vi "Match idot to shot.vi"(8 "error in (no error)":errorcluster, 10 "Idot match record":T1, 11 "Cap Bank Server in":refnum<class "Cap Bank Server.lvclass">) -> (0 "error out":errorcluster, 3 "Cap Bank Server out":refnum<class "Cap Bank Server.lvclass">)   [LabVIEW 2015, in "Cap Bank Server.lvclass"]
uses:
  Cap Bank Server.lvclass
  Idot match record.ctl
  <vilib>/ActorFramework/Actor/Actor.lvclass/Actor.ctl
  <vilib>/ActorFramework/Message Enqueuer/Message Enqueuer.lvclass/Message Enqueuer.ctl
  Mag Lab Measure Controller Messages/Log Status Update Msg/Log Status Update Msg.lvclass/Log Status Update Msg.ctl
  Cap Bank Server Messages/Match idot to shot Msg/Match idot to shot Msg.lvclass/Match idot to shot Msg.ctl
  <vilib>/ActorFramework/Message Enqueuer/Init from Existing Queue.vi
  <vilib>/ActorFramework/Message Enqueuer/Enqueue.vi
  <vilib>/ActorFramework/Message Priority Queue/Priority Enqueue.vi
  <vilib>/ActorFramework/Time-Delayed Send Message/Time-Delayed Send Message.vi
  <vilib>/ActorFramework/Message Enqueuer/Message Enqueuer.lvclass
  Mag Lab Measure Controller Messages/Log Status Update Msg/Log Status Update Msg.lvclass
  Cap Bank Server Messages/Match idot to shot Msg/Match idot to shot Msg.lvclass
  <vilib>/ActorFramework/Actor/Actor.lvclass
  Mag Lab Error Handler/Mag Lab Error Handler.lvclass
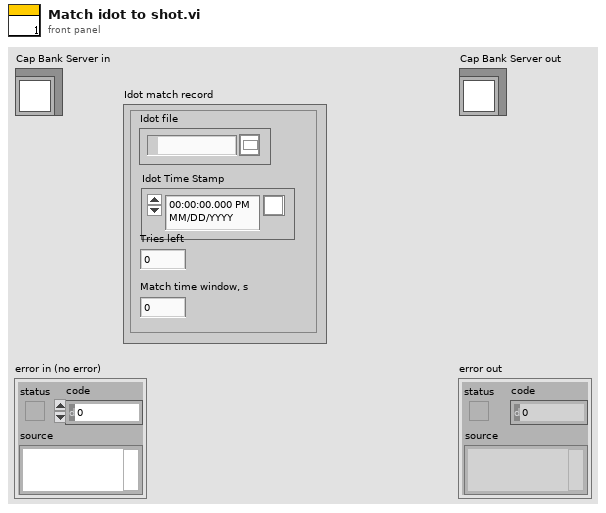
[diagram p1: front panel]
types:
  T1 = typedef "Idot match record.ctl" = cluster{"Idot file":path, "Idot Time Stamp":timestamp, "Tries left":i32, "Match time window, s":dbl}
  T2 = typedef "Shot data.ctl" = cluster{"Shot number":i32, "Time":timestamp, "Magnet ID":string, "User":string, "Cell number":i32, "Requested field":dbl, "Field direction":string, "Number of bank frames":i32, "Crowbar resistance, mOhm":dbl, "Magnet resistance, mOhm":dbl, "Charger voltage, kV":dbl, "Frame voltage, kV":dbl}
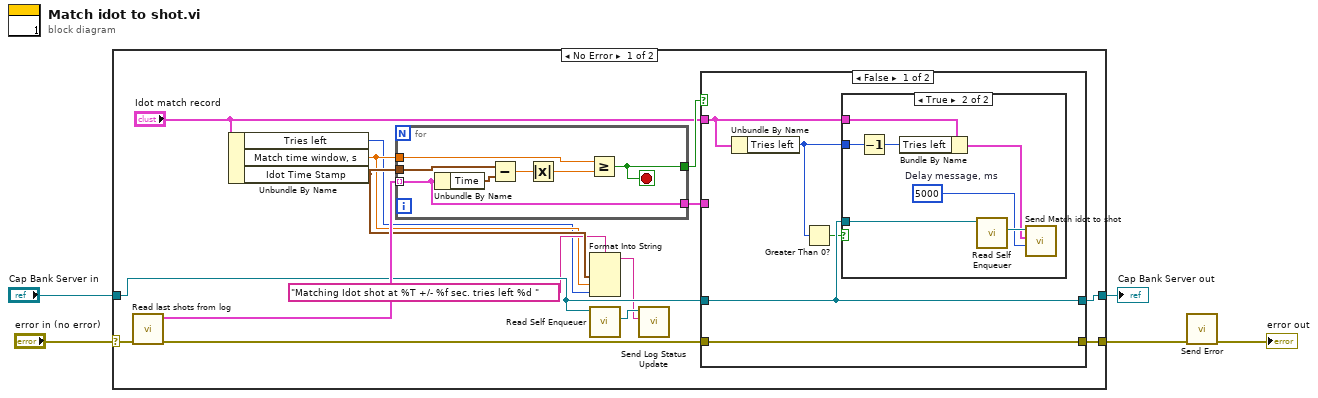
[diagram p0: block diagram]
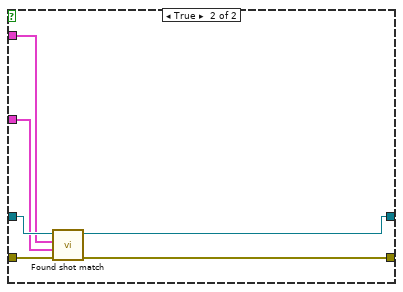
[diagram p3: hidden frame]
diagram:
  n1 = case shown="No Error" "error in (no error)" {
    selector: "error in (no error)" -> [w19 w47]
    tunnel: [w16 w47] -> w2
    tunnel: [w15 w46] -> w3
    tunnel: "Cap Bank Server in" -> [w11 w46]
    frame No Error {
      n2 = call "Read last shots from log.vi"("Error In"=w19) -> ("Error Out"=w17:errorcluster, "Last shots"=w20:T2[])  [unwired: 7 in, 2 out]
      n3 = Unbundle By Name("Idot match record") -> ("Tries left"=w6:i32, "Match time window, s"=w7:dbl, "Idot Time Stamp"=w9:timestamp)
      n4 = for {
        tunnel: w20 -> [w39] mode=indexing
        tunnel: w9 -> [w44]
        tunnel: w7 -> [w41]
        tunnel: [w40] -> w18
        tunnel: [w39] -> w14
        stop <- w40 stop-if-true
        n5 = Unbundle By Name(w39) -> ("Time"=w45:timestamp)
        n6 = Subtract(x=w44, y=w45) -> (x-y=w43:dbl)
        n7 = Absolute Value(x=w43) -> (abs(x)=w42:dbl)
        n8 = Greater Or Equal?(x=w41, y=w42) -> (x >= y?=w40:bool)
      }
      n9 = Format Into String(format string="Matching Idot shot at %T +/- %f sec. tries left %d " ("Status"), w9, w7, w6) -> (resulting string=w10:string)  [unwired: 2 in, 1 out]
      n10 = call <vilib>:"Read Self Enqueuer.vi"("Actor"=w11) -> ("Self Enqueuer"=w12:refnum<class "Message Enqueuer.lvclass">)  [unwired: 10 in]
      n11 = call "Send Log Status Update.vi"("Status"=w10, "Message Enqueuer"=w12) -> ()  [unwired: 8 in, 2 out]
      n12 = case shown="False" w18 {
        tunnel: w17 -> [w25 w38]
        tunnel: [w25 w37] -> w16
        tunnel: w11 -> [w24 w36]
        tunnel: [w24 w35] -> w15
        tunnel: w14 -> [_ w34]
        tunnel: "Idot match record" -> [w23 w33]
        frame False {
          n13 = Unbundle By Name(w23) -> ("Tries left"=w21:i32)
          n14 = Greater Than 0?(x=w21) -> (x > 0?=w22:bool)
          n15 = case shown="True" w22 {
            tunnel: w24 -> [_ w32]
            tunnel: w23 -> [_ w29]
            tunnel: w21 -> [_ w26]
            frame False {
              # "stop trying, let it be"
            }
            frame True {
              w30 = 5000  # Delay message, ms
              n16 = Decrement(x=w26) -> (x-1=w27:i32)
              n17 = Bundle By Name(cluster=w29, "Tries left"=w27) -> (w28:T1)
              n18 = call <vilib>:"Read Self Enqueuer.vi"("Actor"=w32) -> ("Self Enqueuer"=w31:refnum<class "Message Enqueuer.lvclass">)  [unwired: 10 in]
              n19 = call "Send Match idot to shot.vi"("Delay message, ms"=w30, "Idot match record"=w28, "Message Enqueuer"=w31) -> ()  [unwired: 7 in, 2 out]
            }
          }
        }
        frame True {
          n20 = call "Found shot match.vi"("error in (no error)"=w38, "Shot data"=w34, "Idot match record"=w33, "Cap Bank Server in"=w36) -> ("error out"=w37:errorcluster, "Cap Bank Server out"=w35:refnum<class "Cap Bank Server.lvclass">)  [unwired: 6 in]
        }
      }
    }
    frame Error {
    }
  }
  "Cap Bank Server out" <- w3
  n21 = call "Send Error.vi"("error in (no error)"=w2) -> ("error out"=→"error out":errorcluster)  [unwired: 9 in, 1 out]
